vi "subExportDependencies.vi"(8 "error in (no error)":errorcluster, 11 "ILabVIEWItem in":refnum<class "ILabVIEWItem.lvclass">) -> (0 "error out":errorcluster, 1 "Links":T1, 3 "ILabVIEWItem out":refnum<class "ILabVIEWItem.lvclass">)   [LabVIEW 2020, in "DefaultExtensions.lvlib" / "CGrapherDGML.lvclass"]
uses:
  CGrapherDGML.lvclass
  obj/Addons/LabVIEWObjectInterfaces.lvlibp/LabVIEWObjectInterfaces/ILabVIEWItem/ILabVIEWItem.lvclass
  obj/Addons/LabVIEWItem.lvlibp/LabVIEWItem/CLabVIEWItem/ConnectionSet.ctl
  obj/Addons/LabVIEWItem.lvlibp/LabVIEWItem/CLabVIEWItem/CLabVIEWItem.lvclass
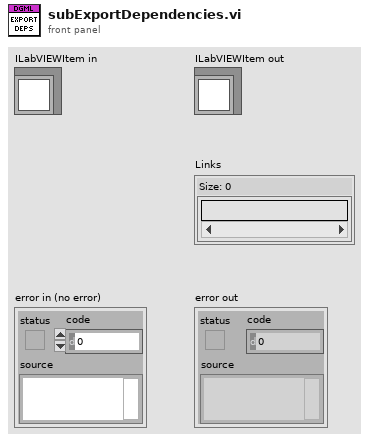
[diagram p1: front panel]
types:
  T1 = typedef "LabVIEWItem.lvlibp/CLabVIEWItem.lvclass/ConnectionSet.ctl" = set{string}
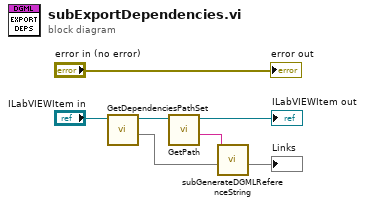
[diagram p0: block diagram]
diagram:
  n1 = call-dynamic "GetDependenciesPathSet.vi"("ILabVIEWItem in"="ILabVIEWItem in") -> ("Dependencies"=w1:set{string}, "ILabVIEWItem out"=w3:refnum<class "ILabVIEWItem.lvclass">)  [unwired: 8 in, 1 out]
  n2 = call-dynamic "GetPath.vi"("ILabVIEWItem in"=w3) -> ("Path"=w5:string, "ILabVIEWItem out"=→"ILabVIEWItem out":refnum<class "ILabVIEWItem.lvclass">)  [unwired: 8 in, 1 out]
  n3 = call "subGenerateDGMLReferenceString.vi"("References"=w1, "Source"=w5) -> ("Links"=→"Links":T1)  [unwired: 9 in]
  "error out" <- "error in (no error)"
